vi "GetImage.vi"(0 "XRef":T5, 1 "State In":T3) -> (14 "Image":T2, 15 "Fatal Error Out":T1)   [LabVIEW 2015, in "LVJSON.lvlib" / "Get Object Parameters.xnode"]
uses:
  Get Object Parameters.xnode
  <vilib>/XNodeSupport/XNodeXNodeRef.ctl
  State.ctl
  Parameter.ctl
  <vilib>/XNodeSupport/XNodeImage.ctl
  <vilib>/XNodeSupport/XNodeErrorCluster.ctl
  Shared/Shared.lvlib
  <vilib>/XNodeSupport/NI_XNodeSupport.lvlib
panel:
  in  "picture":picture
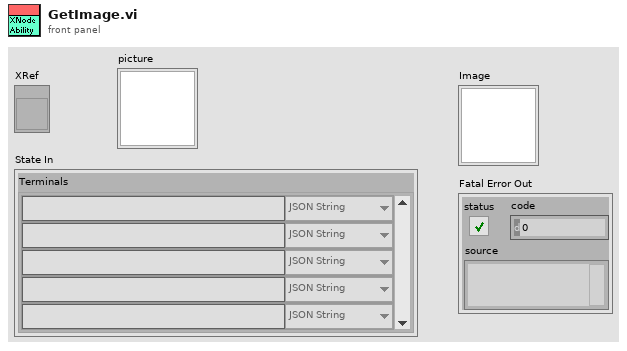
[diagram p1: front panel]
types:
  T1 = typedef "NI_XNodeSupport.lvlib/XNodeErrorCluster.ctl" = errorcluster
  T2 = typedef "NI_XNodeSupport.lvlib/XNodeImage.ctl" = picture
  T3 = typedef "LVJSON.lvlib/Get Object Parameters.xnode/State.ctl" = cluster{"Terminals":T4[]}
  T4 = typedef "LVJSON.lvlib/Shared.lvlib/Parameter.ctl" = cluster{"Parameter Name":string, "JSON Type":enum16{"JSON String", "JSON Numeric", "JSON Boolean", "JSON", "JSON Object", "JSON Array", "String Value", "Numeric Value", "Boolean Value"}}
  T5 = typedef "NI_XNodeSupport.lvlib/XNodeXNodeRef.ctl" = refnum<vi>
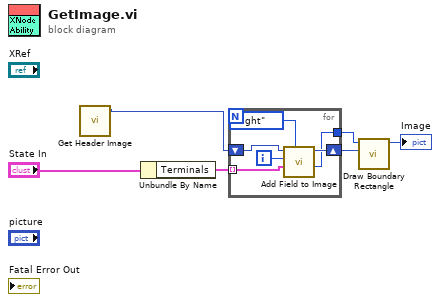
[diagram p0: block diagram]
diagram:
  n1 = call "Get Header Image.vi"() -> ("new picture"=w1:picture)  [unwired: 11 in]
  n2 = Unbundle By Name("State In") -> ("Terminals"=w5:T4[])
  n3 = for {
    shift-right: [w12] -> w4
    shift-left: w1 -> [w11]
    tunnel: w5 -> [w9] mode=indexing
    tunnel: [w8] -> w3
    i -> [w10]
    n4 = call "Add Field to Image.vi"("Justification"=enum16{"Left", "Center", "Right"}."Right", "Terminal Info"=w9, "location"=w10, "picture"=w11) -> ("y"=w8:i16, "new picture"=w12:picture)  [unwired: 6 in]
  }
  n5 = call "Draw Boundary Rectangle.vi"("new picture in"=w4, "y"=w3) -> ("new picture out"=→"Image":picture)  [unwired: 9 in]
